vi "MDrive_Data_Collection(example) test.vi"() -> ()   [LabVIEW 2010]
uses:
  Documents/takada/Labview/FPGA_Batch_1_5/Batch_main Folder/host-subvis/ATMDelayLine/Drivers/Set Parameter.ctl
  Documents/takada/Labview/FPGA_Batch_1_5/Batch_main Folder/host-subvis/ATMDelayLine/Drivers/Get Parameter.ctl
panel:
  out "Position  Graph":dbl[][](graph)
  out "Cycle Time":dbl
  out "Elapsed Time":u32
  in  "VM Setpoint":string="1000000"
  in  "VI Setpoint":string="100000"
  out "Velocity Graph":i32[](graph)
  in  "Move Position":string="512000"
  in  "Decel Setpoint":string="1000000"
  in  "Accel Setpoint":string="1000000"
  in  "Com Port":refnum<visa-resource-name>="COM3"
  in  "baud rate":u32=9600
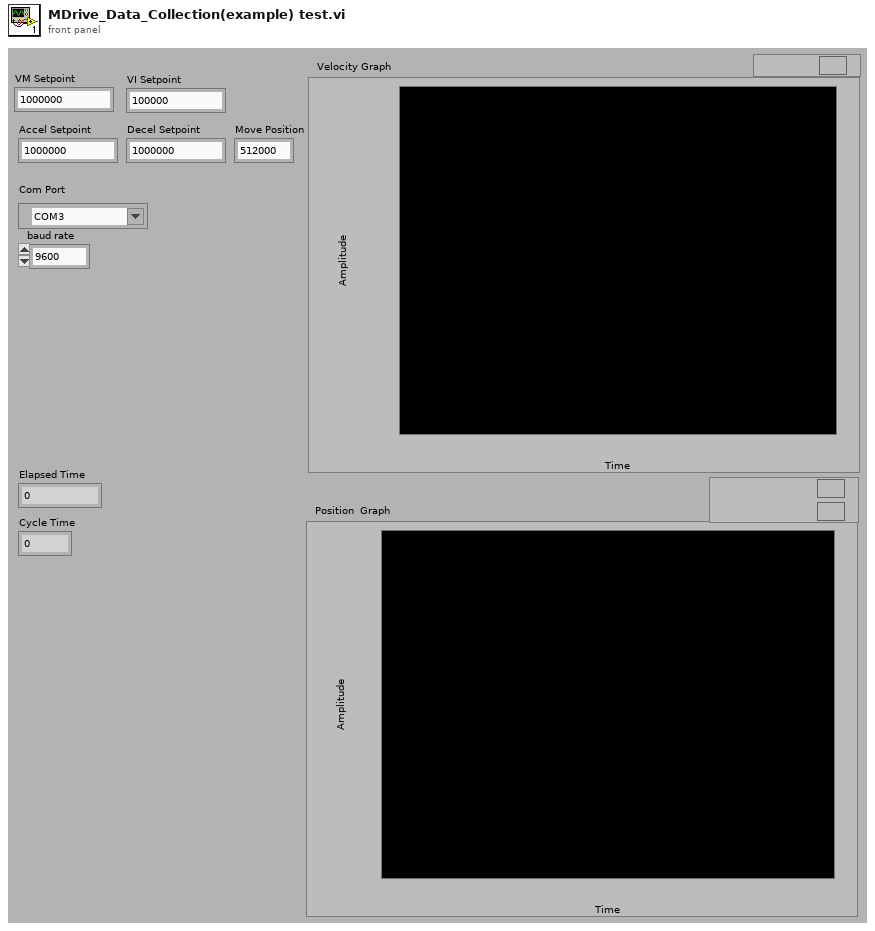
[diagram p1: front panel]
types:
  T1 = typedef "Get Parameter.ctl" = enum16{"Acceleration (A)", "Baud Rate (BD)", "Busy Flag (BY)", "Counter 1 (C1)", "Counter 2 (C2)", "Check Sum Enable (CK)", "Clock Mode (CM)", "Clock Mode Ratio (CR)", "Clock Mode Out Step Width (CW)", "Deceleration (D)", "Digital Filtering, Input 1 (D1)", "Digital Filtering, Input 2 (D2)", "Digital Filtering, Input 3 (D3)", "Digital Filtering, Input 4 (D4)", "Digital Filtering, Input 5 (D5)", "Digital Filtering, Input 9 (D9)", "Digital Filtering, Input 10 (D10)", "Digital Filtering, Input 11 (D11)", "Digital Filtering, Input 12 (D12)", "Deadband (DB)", "Enable/Disable Drive (DE)", "Device Name (DN)", "End Program Execution (E)", "Encoder Function Enable (EE)", "Encoder Lines (EL)", "Error Flag (EF)", "Error Variable (ER)", "Echo Mode (EM)", "Escape (ES)", "Execute Program at Address (EX)", "Hold Current (HC)", "Hold Current Delay Time (HI)", "Input 1 (I1)", "Input 2 (I2)", "Input 3 (I3)", "Input 4 (I4)", "Input 5 Analog (I5)", "Input 6 Encoder Index (I6)", "Input 9 (I9)", "Input 10 (I10)", "Input 11 (I11)", "Input 12 (I12)", "Input Low Byte (1-4) (IL)", "Input High Byte (9-12) (IH)", "Inputs Total (1-4,9-12) (IN)", "Internal Temperature (IT)", "Jog Enable (JE)", "Limit Stop Mode (LM)", "MicroStepping Select (MS)", "Motor Settling Delay Time (MT)", "Moving Flag (MV)", "Output 1 (O1)", "Output 2 (O2)", "Output 3 (O3)", "Output 4 (O4)", "Output 9 (O9)", "Output 10 (O10)", "Output 11 (O11)", "Output 12 (O12)", "Output High Byte (9-12) (OH)", "Output Low Byte (1-4) (OL)", "Output Total (1-4 and 9-12) (OT)", "Position Captured at Trip (PC)", "Position Maintenance (PM)", "Part Number (PN)", "Party Mode (PY)", "Register 1 (R1)", "Register 2 (R2)", "Register 3 (R3)", "Register 4 (R4)", "Run Current (RC)", "Serial Number (SN)", "Stall Flag (ST)", "Stall Factor (SF)", "Stall Mode Set (SM)", "User Variables (UV)", "Velocity (V)", "Velocity Changing Flag (VC)", "Velocity Initial (VI)", "Version, Firmware (VR)", "Velocity Maximum (VM)"}
  T2 = typedef "Set Parameter.ctl" = enum16{"Acceleration (A)", "Baud Rate (BD)", "Counter 1 (C1)", "Counter 2 (C2)", "Control C Software Reset (CE)", "Check Sum Enable (CK)", "Clock Mode (CM)", "Clock Mode Ratio (CR)", "Clock Mode Out Step Width (CW)", "Deceleration (D)", "Digital Filtering, Input 1 (D1)", "Digital Filtering, Input 2 (D2)", "Digital Filtering, Input 3 (D3)", "Digital Filtering, Input 4 (D4)", "Digital Filtering, Input 5 (D5)", "Digital Filtering, Input 9 (D9)", "Digital Filtering, Input 10 (D10)", "Digital Filtering, Input 11 (D11)", "Digital Filtering, Input 12 (D12)", "Deadband (DB)", "Decrement Variable (DC)", "Enable/Disable Drive (DE)", "Device Name (DN)", "End Program Execution (E)", "Encoder Function Enable (EE)", "Encoder Lines (EL)", "Echo Mode (EM)", "Escape (ES)", "Execute Program at Address (EX)", "Hold (H)", "Hold Current (HC)", "Hold Current Delay Time (HI)", "Home to Encoder Index (HM)", "Home to Home Switch (HT)", "Increment Variable (IC)", "Initialize Parameters to NVM (IP)", "Input into Variable (IV)", "Jog Enable (JE)", "Limit Stop Mode (LM)", "Move Absolute (MA)", "Move Relative (MR)", "MicroStepping Select (MS)", "Motor Settling Delay Time (MT)", "Output 1 (O1)", "Output 2 (O2)", "Output 3 (O3)", "Output 4 (O4)", "Output 9 (O9)", "Output 10 (O10)", "Output 11 (O11)", "Output 12 (O12)", "Output High Byte (9-12) (OH)", "Output Low Byte (1-4) (OL)", "Output Total (1-4 and 9-12) (OT)", "Position Maintenance (PM)", "Party Mode (PY)", "Register 1 (R1)", "Register 2 (R2)", "Register 3 (R3)", "Register 4 (R4)", "Run Current (RC)", "Stall Factor (SF)", "Slew (SL)", "Stall Mode Set (SM)", "Upgrade Firmware (UG)", "Velocity Initial (VI)", "Velocity Maximum (VM)"}
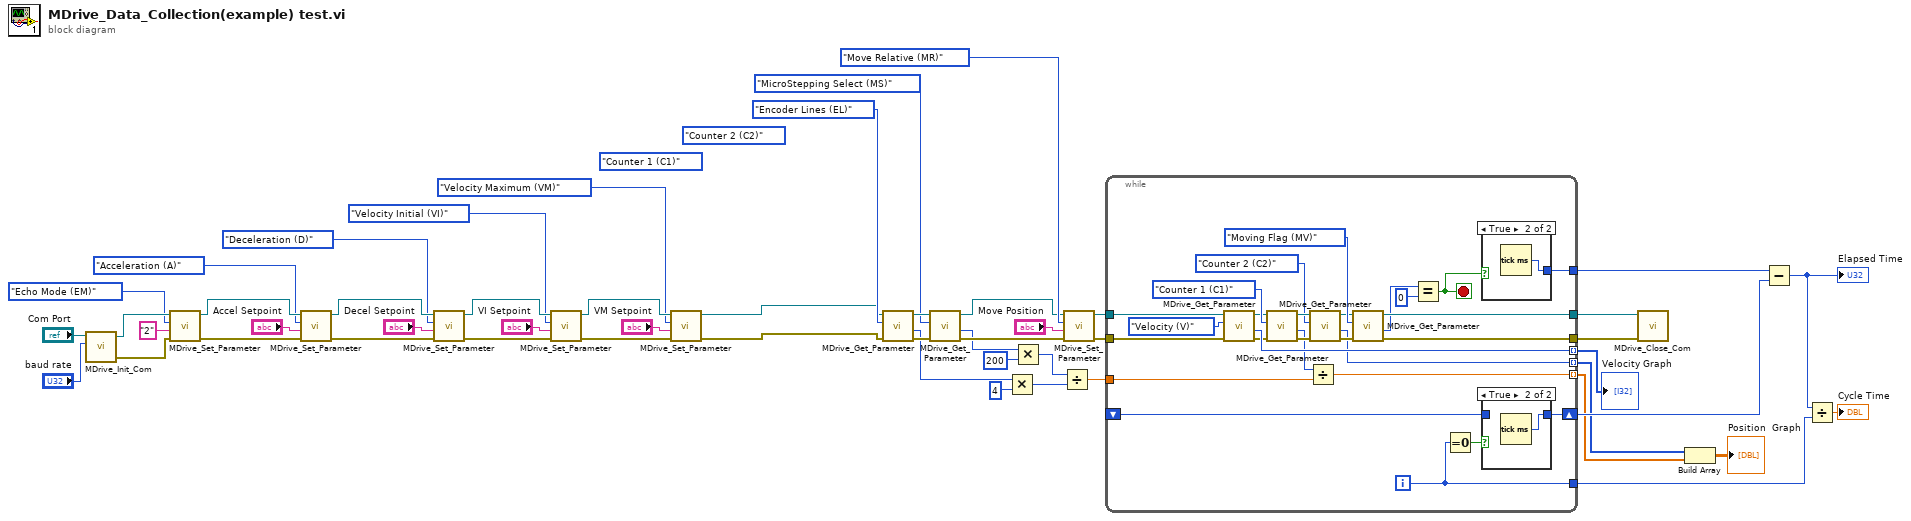
[diagram p0: block diagram]
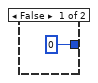
[diagram p2: hidden frame]
diagram:
  (unwired) Set_Parameter."Counter 2 (C2)" ("Set Parameter")
  (unwired) Set_Parameter."Counter 1 (C1)" ("Set Parameter")
  n1 = call "MDrive_Init_Com.vi"("VISA resource name"="Com Port", "baud rate"="baud rate") -> ("VISA resource name out"=w29:refnum<visa-resource-name>, "error out"=w26:errorcluster)  [unwired: 5 in]
  n2 = call "MDrive_Set_Parameter.vi"("error out 2"=w26, "Parameter Setpoint"="2", "Set Parameter"=Set_Parameter."Echo Mode (EM)", "VISA resource name out 2"=w29) -> ("error out"=w30:errorcluster, "VISA resource name out"=w31:refnum<visa-resource-name>)  [unwired: 1 in, 1 out]
  n3 = call "MDrive_Set_Parameter.vi"("error out 2"=w30, "Parameter Setpoint"="Accel Setpoint", "Set Parameter"=Set_Parameter."Acceleration (A)", "VISA resource name out 2"=w31) -> ("error out"=w47:errorcluster, "VISA resource name out"=w49:refnum<visa-resource-name>)  [unwired: 1 in, 1 out]
  n4 = call "MDrive_Set_Parameter.vi"("error out 2"=w47, "Parameter Setpoint"="Decel Setpoint", "Set Parameter"=Set_Parameter."Deceleration (D)", "VISA resource name out 2"=w49) -> ("error out"=w41:errorcluster, "VISA resource name out"=w42:refnum<visa-resource-name>)  [unwired: 1 in, 1 out]
  n5 = call "MDrive_Set_Parameter.vi"("error out 2"=w41, "Parameter Setpoint"="VI Setpoint", "Set Parameter"=Set_Parameter."Velocity Initial (VI)", "VISA resource name out 2"=w42) -> ("error out"=w38:errorcluster, "VISA resource name out"=w39:refnum<visa-resource-name>)  [unwired: 1 in, 1 out]
  n6 = call "MDrive_Set_Parameter.vi"("error out 2"=w38, "Parameter Setpoint"="VM Setpoint", "Set Parameter"=Set_Parameter."Velocity Maximum (VM)", "VISA resource name out 2"=w39) -> ("error out"=w1:errorcluster, "VISA resource name out"=w2:refnum<visa-resource-name>)  [unwired: 1 in, 1 out]
  n7 = call "MDrive_Get_Parameter.vi"("error in"=w1, "Get Parameter"=Get_Parameter."Encoder Lines (EL)", "VISA resource name in"=w2) -> ("error out"=w19:errorcluster, "Parameter Data Numeric"=w14:i32, "VISA resource name out"=w20:refnum<visa-resource-name>)  [unwired: 1 in, 1 out]
  n8 = call "MDrive_Get_Parameter.vi"("error in"=w19, "Get Parameter"=Get_Parameter."MicroStepping Select (MS)", "VISA resource name in"=w20) -> ("error out"=w17:errorcluster, "Parameter Data Numeric"=w12:i32, "VISA resource name out"=w18:refnum<visa-resource-name>)  [unwired: 1 in, 1 out]
  n9 = Multiply(x=w14, y=4) -> (x*y=w9:i32)
  n10 = Multiply(x=w12, y=200) -> (x*y=w10:i32)
  n11 = Divide(x=w10, y=w9) -> (x/y=w8:dbl)
  n12 = call "MDrive_Set_Parameter.vi"("error out 2"=w17, "Parameter Setpoint"="Move Position", "Set Parameter"=Set_Parameter."Move Relative (MR)", "VISA resource name out 2"=w18) -> ("error out"=w45:errorcluster, "VISA resource name out"=w44:refnum<visa-resource-name>)  [unwired: 1 in, 1 out]
  n13 = while {
    tunnel: w45 -> [w79]
    tunnel: w44 -> [w78]
    tunnel: [w77] -> w4
    tunnel: [w76] -> w3
    tunnel: [w67] -> w43 mode=indexing
    tunnel: [w74] -> w35
    tunnel: [w73] -> w33
    shift-right: [w71] -> w36
    shift-left: _ -> [w70]
    tunnel: w8 -> [w57]
    tunnel: [w54] -> w6 mode=indexing
    tunnel: [w53] -> w5 mode=indexing
    i -> [w73]
    stop <- w66 stop-if-true
    n14 = call "MDrive_Get_Parameter.vi"("error in"=w79, "Get Parameter"=Get_Parameter."Velocity (V)", "VISA resource name in"=w78) -> ("error out"=w60:errorcluster, "Parameter Data Numeric"=w67:i32, "VISA resource name out"=w61:refnum<visa-resource-name>)  [unwired: 1 in, 1 out]
    n15 = call "MDrive_Get_Parameter.vi"("error in"=w60, "Get Parameter"=Get_Parameter."Counter 1 (C1)", "VISA resource name in"=w61) -> ("error out"=w64:errorcluster, "Parameter Data Numeric"=w58:i32, "VISA resource name out"=w63:refnum<visa-resource-name>)  [unwired: 1 in, 1 out]
    n16 = Divide(x=w58, y=w57) -> (x/y=w53:dbl)
    n17 = call "MDrive_Get_Parameter.vi"("error in"=w64, "Get Parameter"=Get_Parameter."Counter 2 (C2)", "VISA resource name in"=w63) -> ("error out"=w56:errorcluster, "Parameter Data Numeric"=w54:i32, "VISA resource name out"=w55:refnum<visa-resource-name>)  [unwired: 1 in, 1 out]
    n18 = call "MDrive_Get_Parameter.vi"("error in"=w56, "Get Parameter"=Get_Parameter."Moving Flag (MV)", "VISA resource name in"=w55) -> ("error out"=w76:errorcluster, "Parameter Data Numeric"=w69:i32, "VISA resource name out"=w77:refnum<visa-resource-name>)  [unwired: 1 in, 1 out]
    n19 = Equal?(x=w69, y=i16 0) -> (x = y?=w66:bool)
    n20 = Equal To 0?(x=w73) -> (x = 0?=w72:bool)
    n21 = case shown="True" w66 {
      tunnel: [u32 0 ("millisecond timer value") w81] -> w74
      frame False {
      }
      frame True {
        n22 = Tick Count (ms)() -> (millisecond timer value=w81:u32)
      }
    }
    n23 = case shown="True" w72 {
      tunnel: [w82 w83] -> w71
      tunnel: w70 -> [w82 _]
      frame False {
      }
      frame True {
        n24 = Tick Count (ms)() -> (millisecond timer value=w83:u32)
      }
    }
  }
  "Velocity Graph" <- w43
  n25 = call "MDrive_Close_Com.vi"("error out"=w3, "VISA resource name out"=w4) -> ()  [unwired: 2 in]
  n26 = Build Array(w6, w5) -> (→"Position  Graph":dbl[][])
  n27 = Subtract(x=w35, y=w36) -> (x-y=w34:u32)
  "Elapsed Time" <- w34
  n28 = Divide(x=w34, y=w33) -> (x/y=→"Cycle Time":dbl)
